vi "Create evenly spaced array.vi"(1 "Final":dbl=5.4 format="%_6g", 2 "Nbr point":dbl=0.1 format="%_6g", 3 "Initial":dbl=0.7 format="%_6g") -> (0 "Array out":dbl[](array[numeric])=[0.7, 0.7999999999999999, 0.8999999999999999, 1.0, 1.1, 1.2, 1.3, 1.4, 1.5, 1.6, 1.7, 1.8, 1.9000000000000001, 2.0, 2.1, 2.2, 2.3, 2.4000000000000004, 2.5, 2.6, 2.7, 2.8, 2.9000000000000004, 3.0, 3.1000000000000005, 3.2, 3.3, 3.4000000000000004, 3.5, 3.6000000000000005, 3.7, 3.8, 3.9000000000000004, 4.0, 4.1000000000000005, 4.2, 4.3, 4.4, 4.5, 4.6000000000000005, 4.7, 4.800000000000001, 4.9, 5.0, 5.1000000000000005, 5.2, 5.300000000000001])   [LabVIEW 2015]
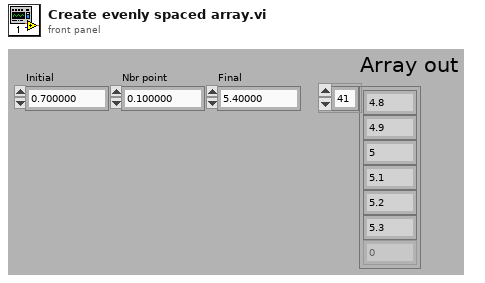
[diagram p1: front panel]
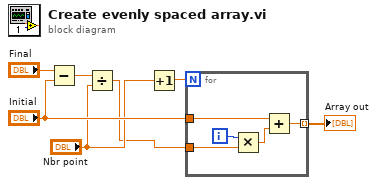
[diagram p0: block diagram]
diagram:
  n1 = Subtract(x="Final", y="Initial") -> (x-y=w7:dbl)
  n2 = Divide(x=w7, y="Nbr point") -> (x/y=w1:dbl)
  n3 = Increment(x="Nbr point") -> (x+1=w3:dbl)
  n4 = for {
    N: w3 -> [_]
    tunnel: w1 -> [w11]
    tunnel: "Initial" -> [w10]
    tunnel: [w8] -> w6 mode=indexing
    i -> [w12]
    n5 = Multiply(x=w12, y=w11) -> (x*y=w9:dbl)
    n6 = Add(x=w10, y=w9) -> (x+y=w8:dbl)
  }
  "Array out" <- w6
